vi "Load HW Database (Core).vi"(8 "error in":errorcluster, 10 "hw db path in":path, 11 "Node Ptr":u64) -> (0 "error out":errorcluster)   [LabVIEW 2020, in "Ballard 1553 System Explorer.lvlib"]
uses:
  Ballard 1553 System Explorer.lvlib
  <vilib>/NI VeriStand/Custom Device API/Custom Device API.lvlib
  <vilib>/NI VeriStand/Custom Device API/Get Item Property (Path).vi
  <vilib>/NI VeriStand/Custom Device Tools/Custom Device Utility Library/Custom Device Utility Library.lvlib
  <vilib>/NI VeriStand/Custom Device API/Set Item Property (Path).vi
  <vilib>/NI VeriStand/Custom Device API/Set Item Property (String).vi
  Shared/Controls and Global/Global.vi
  Shared/Ballard 1553 Shared.lvlib
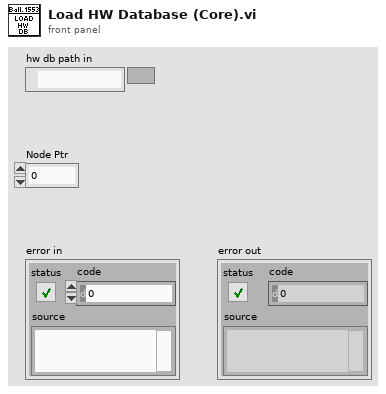
[diagram p1: front panel]
types:
  T1 = typedef "Custom Device API.lvlib/Custom Device Item Ref.ctl" = u64
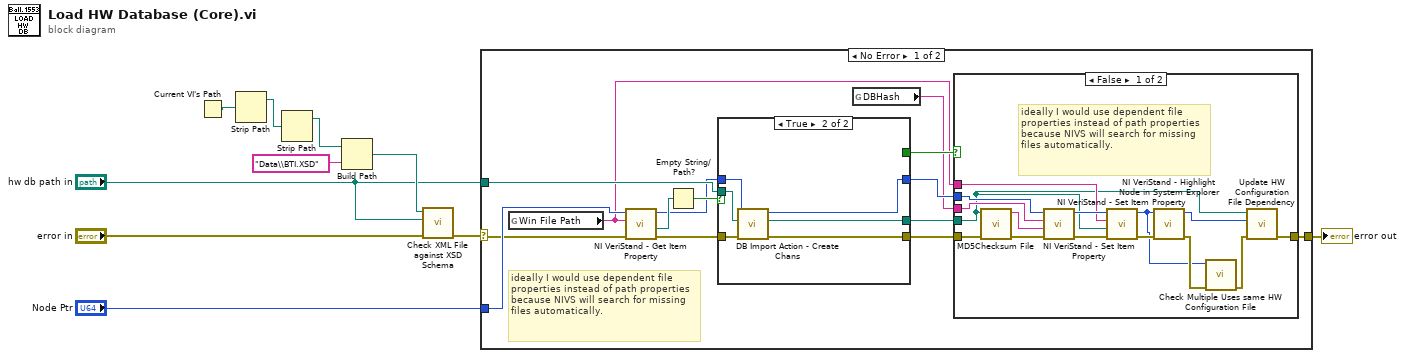
[diagram p0: block diagram]
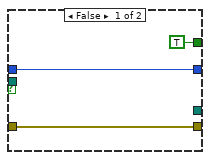
[diagram p3: hidden frame]
diagram:
  n1 = Current VI's Path() -> (path=w8:path)
  n2 = Strip Path(path=w8) -> (stripped path=w7:path)  [unwired: 1 out]
  n3 = Strip Path(path=w7) -> (stripped path=w6:path)  [unwired: 1 out]
  n4 = Build Path(base path=w6, name or relative path="Data\\BTI.XSD") -> (appended path=w9:path)
  n5 = call "Check XML File against XSD Schema.vi"("error in (no error)"="error in", "XML Configuration File Path"="hw db path in", "XML Schema File Path"=w9) -> ("error IO"=w3:errorcluster)  [unwired: 8 in]
  n6 = case shown="No Error" w3 {
    selector: w3 -> [w13 w50]
    tunnel: [w21 w50] -> w1
    tunnel: "Node Ptr" -> [w20 _]
    tunnel: "hw db path in" -> [w17 _]
    frame No Error {
      # "ideally I would use dependent file properties instead of path properties because NIVS will search for missing files automatically."
      n7 = global read "Global.vi" "Win File Path"() -> (w12:string)
      n8 = call-poly <vilib>:"NI VeriStand - Get Item Property.vi"("error in (no error)"=w13, "Property Name"=w12, "Item Ref in"=w20) -> ("error out"=w14:errorcluster, "Value"=w18:path, "Item Ref out"=w15:T1)  [unwired: 5 in, 1 out]
      n9 = Empty String/Path?(string/path=w18) -> (empty?=w16:bool)
      n10 = case shown="True" w16 {
        tunnel: [w43 w49] -> w24
        tunnel: [w42 w48] -> w23
        tunnel: [_ w47] -> w22
        tunnel: w14 -> [w43 w46]
        tunnel: [TRUE ("Cancelled?") _] -> w19
        tunnel: w17 -> [_ w45]
        tunnel: w15 -> [w42 w44]
        frame False {
        }
        frame True {
          n11 = call "DB Import Action - Create Chans.vi"("error in (no error)"=w46, "selected path"=w45, "Node Ptr"=w44) -> ("error out"=w49:errorcluster, "selected path out"=w47:path, "Node Ptr dup"=w48:u64)  [unwired: 6 in]
        }
      }
      n12 = global read "Global.vi" "DBHash"() -> (w11:string)
      n13 = case shown="False" w19 {
        tunnel: w24 -> [w33 w40]
        tunnel: w23 -> [w39 _]
        tunnel: w22 -> [w29 _]
        tunnel: [w30 w40] -> w21
        tunnel: w11 -> [w35 _]
        tunnel: w12 -> [w34 _]
        frame False {
          # "ideally I would use dependent file properties instead of path properties because NIVS will search for missing files automatically."
          n14 = call <vilib>:"MD5Checksum File.vi"("error in (no error)"=w33, "Path"=w29) -> ("error out"=w32:errorcluster, "MD5 message-digest"=w31:string)  [unwired: 8 in]
          n15 = call-poly <vilib>:"NI VeriStand - Set Item Property.vi"("error in (no error)"=w32, "Value"=w31, "Property Name"=w35, "Item Ref in"=w39) -> ("error out"=w36:errorcluster, "Item Ref out"=w37:T1)  [unwired: 5 in, 1 out]
          n16 = call-poly <vilib>:"NI VeriStand - Set Item Property.vi"("error in (no error)"=w36, "Value"=w29, "Property Name"=w34, "Item Ref in"=w37) -> ("error out"=w38:errorcluster, "Item Ref out"=w25:T1)  [unwired: 5 in, 1 out]
          n17 = call <vilib>:"NI VeriStand - Highlight Node in System Explorer.vi"("error in (no error)"=w38, "Item Ref in"=w25) -> ("error out"=w27:errorcluster, "Node Ptr dup"=w28:T1)  [unwired: 8 in]
          n18 = call "Check Multiple Uses same HW Configuration File.vi"("error in (no error)"=w27, "Item Ref in"=w25) -> ("error out"=w26:errorcluster)  [unwired: 9 in]
          n19 = call "Update HW Configuration File Dependency.vi"("error in (no error)"=w26, "Node Ptr dup"=w28, "selected path in"=w29) -> ("error out"=w30:errorcluster)  [unwired: 8 in]
        }
        frame True {
        }
      }
    }
    frame Error {
    }
  }
  "error out" <- w1
